vi "HB_ReadAI.vi"(8 "error in (no error)":errorcluster, 9 "Pin number 0-7":dbl, 10 "Mode":T2=enum."Single Channel", 11 "“HBDeviceRef_in":T1) -> (0 "All ADC raw values":u32[](array[numeric]) format="%012b", 1 "All ADC voltages":dbl[](array[numeric]), 2 "Single Scaled Voltage":dbl, 3 "Single Raw Voltage":u32, 4 "error out":errorcluster, 5 "“HBDeviceRef_out":T1)   [LabVIEW 2016]
uses:
  ReadAI Modes.ctl
  <vilib>/Rock Robotics/WPI/SerialPort/WPI_SerialPortRef.ctl
panel:
  out "Buffer":string
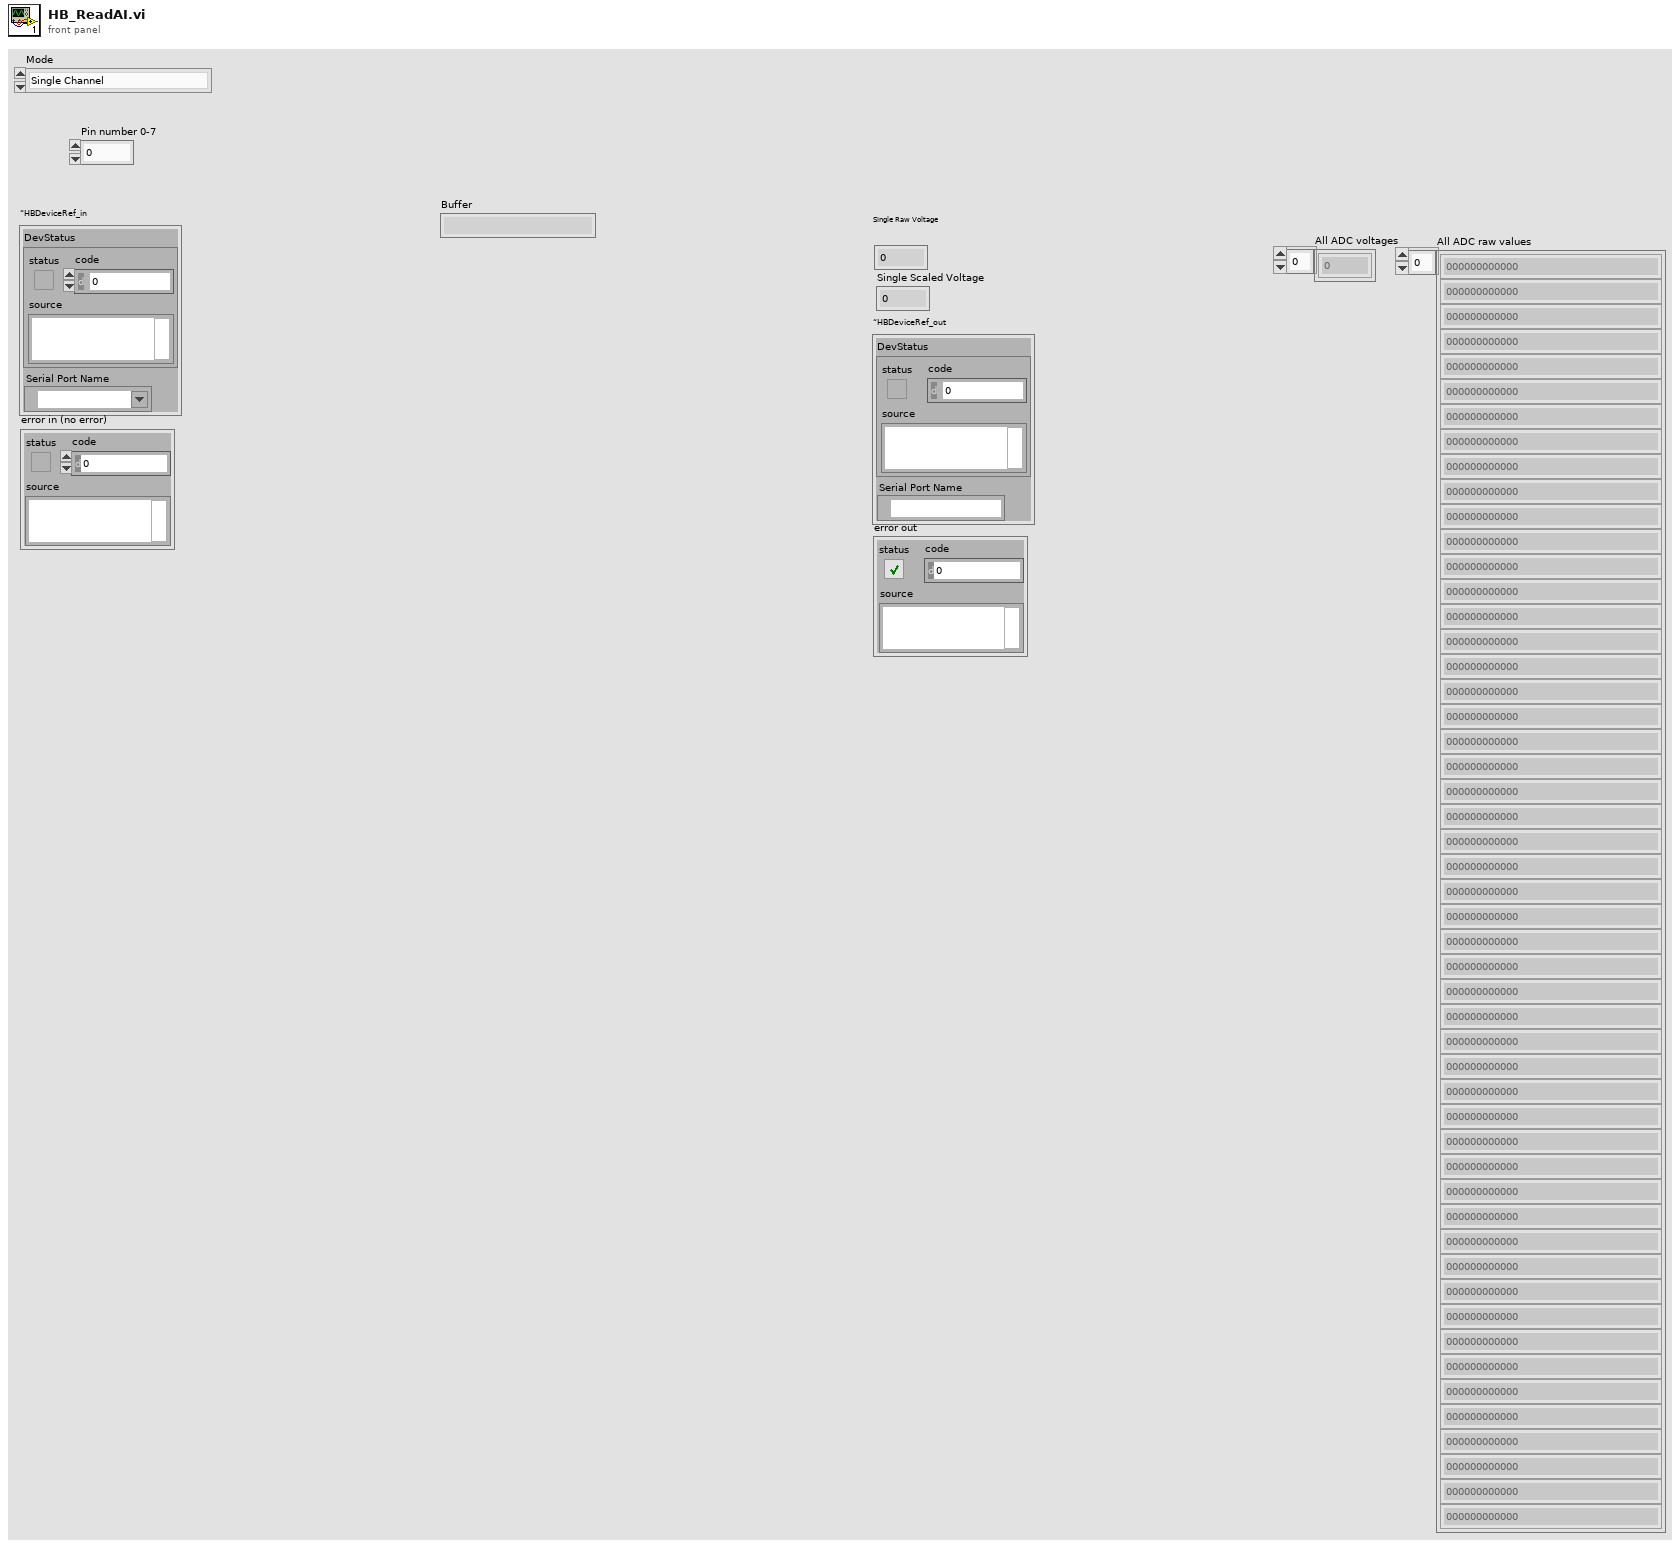
[diagram p1: front panel]
types:
  T1 = typedef "WPI_SerialPortRef.ctl" = cluster{"DevStatus":errorcluster, "Serial Port Name":refnum<visa-resource-name>}
  T2 = typedef "ReadAI Modes.ctl" = enum16{"All Channels", "Single Channel"}
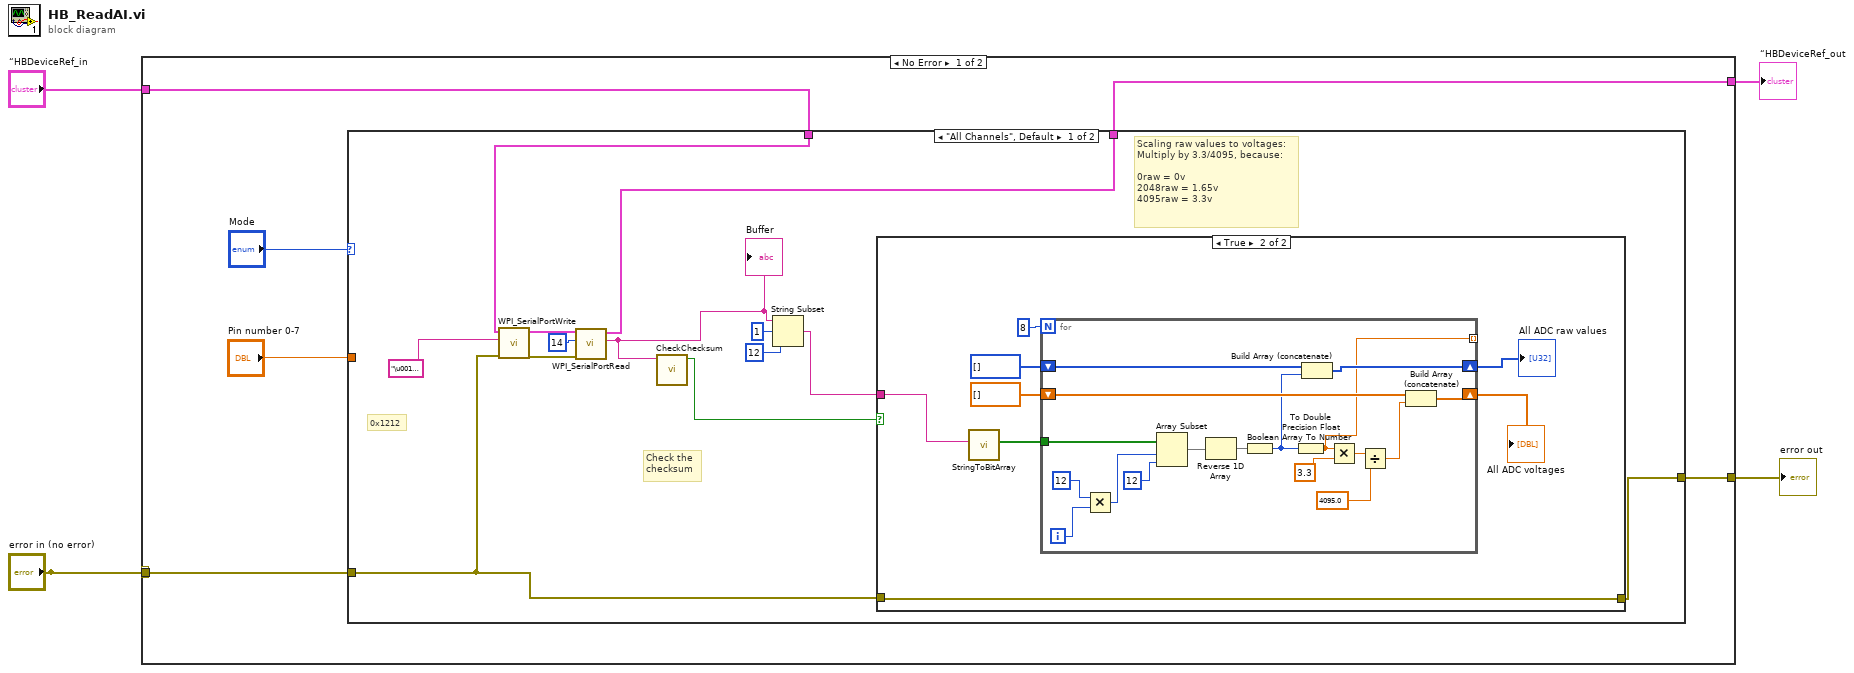
[diagram p0: block diagram]
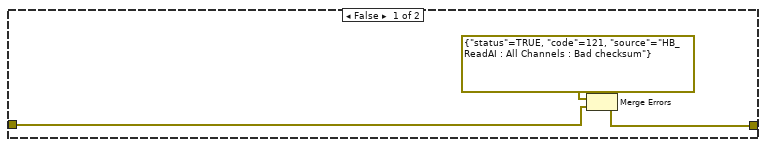
[diagram p2: hidden frame]
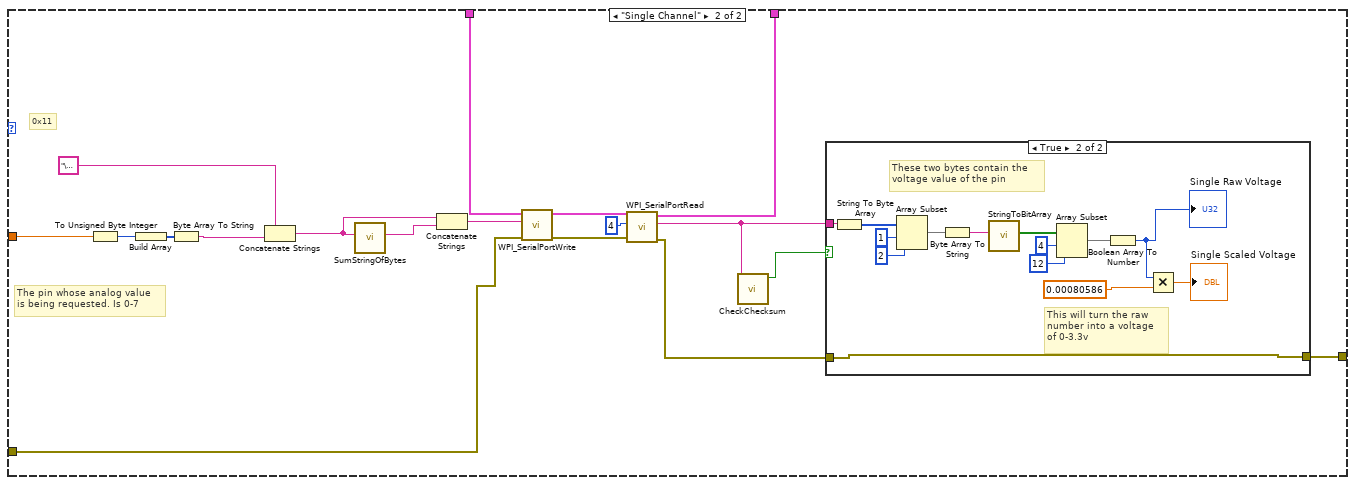
[diagram p3: hidden frame]
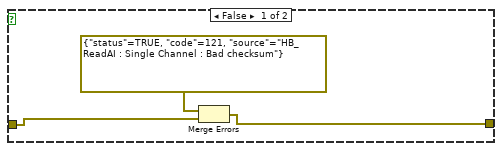
[diagram p4: hidden frame]
diagram:
  n1 = case shown="No Error" "error in (no error)" {
    selector: "error in (no error)" -> [_ w87]
    tunnel: [w9 w87] -> w4
    tunnel: "error in (no error)" -> [w8 _]
    tunnel: "“HBDeviceRef_in" -> [w6 w88]
    tunnel: [w5 w88] -> w2
    frame No Error {
      n2 = case shown="\"All Channels\", Default" "Mode" {
        tunnel: [w14 w56] -> w9
        tunnel: w8 -> [w13 w55]
        tunnel: "Pin number 0-7" -> [_ w54]
        tunnel: w6 -> [w12 w53]
        tunnel: [w11 w52] -> w5
        frame "All Channels", Default {
          # "Scaling raw values to voltages:\nMultiply by 3.3/4095, because:\n\n0raw = 0v\n2048raw = 1.65v\n4095raw = 3.3v"
          # "Check the\nchecksum"
          # "0x1212"
          n3 = call <vilib>:"WPI_SerialPortWrite.vi"("error in (no error)"=w13, "Buffer"="\u0012\u0012", "SerialPortRef"=w12) -> ("error out"=w20:errorcluster, "SerialPortRef"=w19:T1)  [unwired: 6 in, 1 out]
          n4 = call <vilib>:"WPI_SerialPortRead.vi"("error in (no error)"=w20, "Num Bytes to Read"=u32 14, "SerialPortRef"=w19) -> ("Buffer"=w22:string, "SerialPortRef"=w11:T1)  [unwired: 6 in, 1 out]
          "Buffer" <- w22
          n5 = call "CheckChecksum.vi"("String"=w22) -> ("x = y?"=w23:bool)  [unwired: 9 in, 1 out]
          n6 = String Subset(string=w22, offset (0)=1, length (rest)=12 ("length (rest)")) -> (substring=w18:string)
          n7 = case shown="True" w23 {
            tunnel: w18 -> [_ w29]
            tunnel: w13 -> [w25 w34]
            tunnel: [w24 w34] -> w14
            frame False {
              n8 = Merge Errors(errorcluster {"status"=TRUE, "code"=121, "source"="HB_ReadAI : All Channels : Bad checksum"} ("error in"), w25) -> (w24:errorcluster)
            }
            frame True {
              n9 = call "StringToBitArray.vi"("string"=w29) -> ("Array"=w32:bool[])  [unwired: 10 in]
              n10 = for {
                N: 8 -> [_]
                tunnel: w32 -> [w51]
                shift-right: [w47] -> w30
                shift-left: u32[] [] -> [w46]
                shift-right: [w42] -> w27
                shift-left: dbl[] [] -> [w41]
                tunnel: [w35] -> _ mode=indexing
                i -> [w50]
                n11 = Multiply(x=12, y=w50) -> (x*y=w48:i32)
                n12 = Array Subset(array=w51, index=w48, length=12) -> (w44:bool[])
                n13 = Reverse 1D Array(array=w44) -> (reversed array=w43:bool[])
                n14 = Boolean Array To Number(Boolean array=w43) -> (number=w36:u32)
                n15 = To Double Precision Float(number=w36) -> (double precision float=w35:dbl)
                n16 = Build Array (concatenate)(w46, w36) -> (w47:u32[])
                n17 = Multiply(x=w35, y=3.3) -> (x*y=w39:dbl)
                n18 = Divide(x=w39, y=4095.0) -> (x/y=w37:dbl)
                n19 = Build Array (concatenate)(w41, w37) -> (w42:dbl[])
              }
              "All ADC raw values" <- w30
              "All ADC voltages" <- w27
            }
          }
        }
        frame "Single Channel" {
          # "The pin whose analog value\nis being requested. Is 0-7"
          # "0x11"
          n20 = To Unsigned Byte Integer(number=w54) -> (unsigned 8bit integer=w60:u8)
          n21 = Build Array(w60) -> (w63:u8[])
          n22 = Byte Array To String(unsigned byte array=w63) -> (string=w58:string)
          n23 = Concatenate Strings("\u0011" ("Buffer"), w58) -> (w57:string)
          n24 = call "SumStringOfBytes.vi"("String Of Bytes"=w57) -> ("SumAsString"=w62:string)  [unwired: 10 in]
          n25 = Concatenate Strings(w57, w62) -> (w61:string)
          n26 = call <vilib>:"WPI_SerialPortWrite.vi"("error in (no error)"=w55, "Buffer"=w61, "SerialPortRef"=w53) -> ("error out"=w68:errorcluster, "SerialPortRef"=w69:T1)  [unwired: 6 in, 1 out]
          n27 = call <vilib>:"WPI_SerialPortRead.vi"("error in (no error)"=w68, "Num Bytes to Read"=u32 4, "SerialPortRef"=w69) -> ("error out"=w64:errorcluster, "Buffer"=w66:string, "SerialPortRef"=w52:T1)  [unwired: 6 in]
          n28 = call "CheckChecksum.vi"("String"=w66) -> ("x = y?"=w65:bool)  [unwired: 9 in, 1 out]
          n29 = case shown="True" w65 {
            tunnel: w66 -> [_ w74]
            tunnel: w64 -> [w72 w73]
            tunnel: [w70 w73] -> w56
            frame False {
              n30 = Merge Errors(errorcluster {"status"=TRUE, "code"=121, "source"="HB_ReadAI : Single Channel : Bad checksum"} ("error in"), w72) -> (w70:errorcluster)
            }
            frame True {
              # "This will turn the raw \nnumber into a voltage \nof 0-3.3v"
              # "These two bytes contain the \nvoltage value of the pin"
              n31 = String To Byte Array(string=w74) -> (unsigned byte array=w86:u8[])
              n32 = Array Subset(array=w86, index=1, length=2) -> (w83:u8[])
              n33 = Byte Array To String(unsigned byte array=w83) -> (string=w82:string)
              n34 = call "StringToBitArray.vi"("string"=w82) -> ("Array"=w81:bool[])  [unwired: 10 in]
              n35 = Array Subset(array=w81, index=4, length=12) -> (w78:bool[])
              n36 = Boolean Array To Number(Boolean array=w78) -> (number=w77:u32)
              "Single Raw Voltage" <- w77
              n37 = Multiply(x=w77, y=0.00080586) -> (x*y=→"Single Scaled Voltage":dbl)
            }
          }
        }
      }
    }
    frame Error {
    }
  }
  "error out" <- w4
  "“HBDeviceRef_out" <- w2
